vi "DeviceReadArea.vi"(7 "error in (no error)":errorcluster, 8 "Amount":i32, 9 "Address":u16=1, 10 "AreaID":T1(ring), 11 "Handle In":u64[](array[numeric])) -> (1 "Data":u16[](array[numeric]), 2 "Result":i32, 3 "Handle Out":u64[](array[numeric]), 5 "error out":errorcluster)   [LabVIEW 2020, in "SnapMB.lvlib"]
uses:
  SnapMB.lvlib
  windows/snapmb.dll
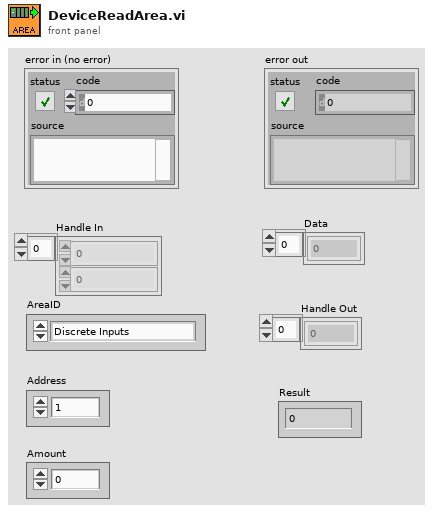
[diagram p1: front panel]
types:
  T1 = enum16{"Discrete Inputs", "Coils", "Input Registers", "Holding Registers"}
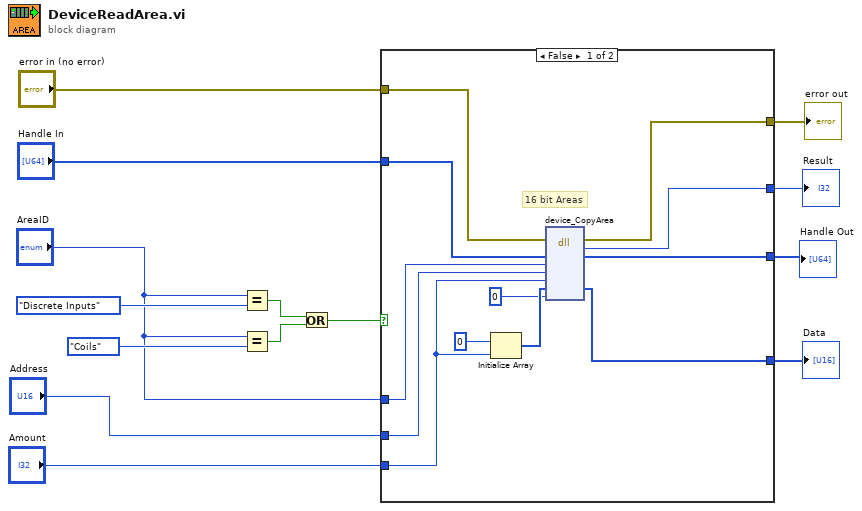
[diagram p0: block diagram]
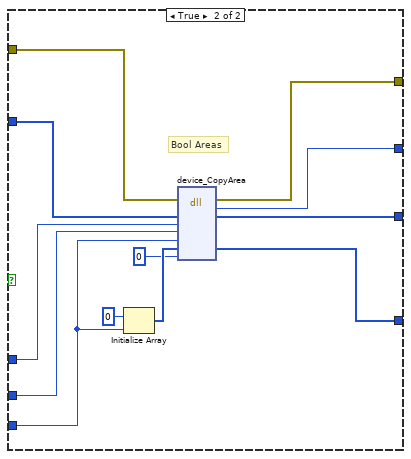
[diagram p2: hidden frame]
diagram:
  n1 = Equal?(x="AreaID", y=T1."Discrete Inputs") -> (x = y?=w12:bool)
  n2 = Equal?(x="AreaID", y=T1."Coils") -> (x = y?=w11:bool)
  n3 = Or(x=w12, y=w11) -> (x .or. y?=w10:bool)
  n4 = case shown="False" w10 {
    tunnel: "Handle In" -> [w26 w27]
    tunnel: "AreaID" -> [w25 w33]
    tunnel: "Amount" -> [w18 w30]
    tunnel: [w24 w35] -> w6
    tunnel: [w23 w36] -> w5
    tunnel: [w22 w37] -> w4
    tunnel: "error in (no error)" -> [w21 w38]
    tunnel: "Address" -> [w19 w32]
    tunnel: [w16 w34] -> w1
    frame False {
      # "16 bit Areas"
      n5 = Initialize Array(u16 0 ("element"), w18) -> (w17:u16[])
      n6 = dll-call lib="D:/SnapMB/LabView/lib/windows/snapmb.dll" fn="device_CopyArea"(error in=w21, "Device"=w26, "AreaID"=w25, "Address"=w19, "Amount"=w18, "Data"=w17, "CopyMode"=0) -> (error out=w22:errorcluster, "Result"=w23:i32, "Device"=w24:u64[], "Data"=w16:u16[])  [unwired: 6 in, 1 out]
    }
    frame True {
      # "Bool Areas"
      n7 = Initialize Array(u8 0 ("element"), w30) -> (w29:u8[])
      n8 = dll-call lib="D:/SnapMB/LabView/lib/windows/snapmb.dll" fn="device_CopyArea"(error in=w38, "Device"=w27, "AreaID"=w33, "Address"=w32, "Amount"=w30, "Data"=w29, "CopyMode"=0) -> (error out=w37:errorcluster, "Result"=w36:i32, "Device"=w35:u64[], "Data"=w34:u8[])  [unwired: 6 in, 1 out]
    }
  }
  "Handle Out" <- w6
  "Result" <- w5
  "error out" <- w4
  "Data" <- w1
